vi "Tell Forward Self.vi"(6 "Msg":refnum<class "Msg.lvclass">, 7 "Actor in":refnum<class "Actor.lvclass">, 9 "Msg DVR":refnum<data-value>) -> (0 "Error out":errorcluster, 5 "Actor out":refnum<class "Actor.lvclass">)   [LabVIEW 2020, in "jettl.lvlib"]
uses:
  jettl.lvlib
  Msg/Msg.lvclass
  Msg Contents/Msg Contents.lvclass
  Actor/Actor.lvclass
  Unified Actor Relation.ctl
  Teller.ctl
  Msg.ctl
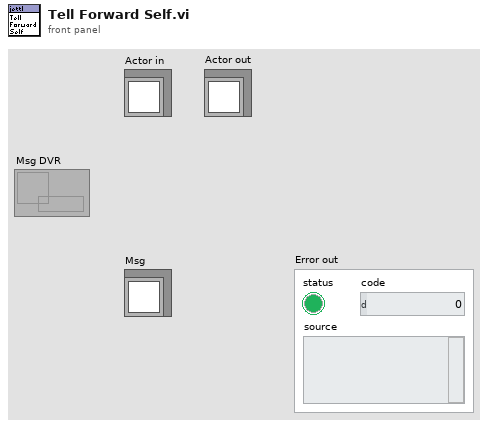
[diagram p1: front panel]
types:
  T1 = typedef "jettl.lvlib/Msg.ctl" = cluster{"Msg":refnum<class "Msg.lvclass">, "Msg Contents":refnum<class "Msg Contents.lvclass">, "Teller":T2}
  T2 = typedef "jettl.lvlib/Teller.ctl" = cluster{"Unified Actor Alias":string, "Unified Actor Relation":T3, "Absolute Time":timestamp, "Relative Time":dbl}
  T3 = typedef "jettl.lvlib/Unified Actor Relation.ctl" = enum16{"Self", "Parent", "Child"}
  T4 = typedef "jettl.lvlib/Unified Actor.ctl" = cluster{"Msgs":T5, "Leaf":bool, "Edge Actors":refnum<class "Actor.lvclass">[], "Mid Actors":refnum<class "Actor.lvclass">[], "Core Actors":refnum<class "Actor.lvclass">[], "Root":bool, "Alias":string, "UID":i32, "Transport":refnum<user-event>, "Address":refnum<event-registration>, "This VI":refnum<vi>}
  T5 = typedef "jettl.lvlib/Msgs.ctl" = cluster{"Inbound":T6, "Outbound":T6, "Implemented":T6, "Tell Init":T6, "Tell Init Self":T6, "Tell Init Parent":T6, "Tell Init Child":T6, "Tell Forward":T6, "Tell Forward Self":T6, "Tell Forward Parent":T6, "Tell Forward Child":T6}
  T6 = typedef "jettl.lvlib/Msg Set.ctl" = set{refnum<class "Msg.lvclass">}
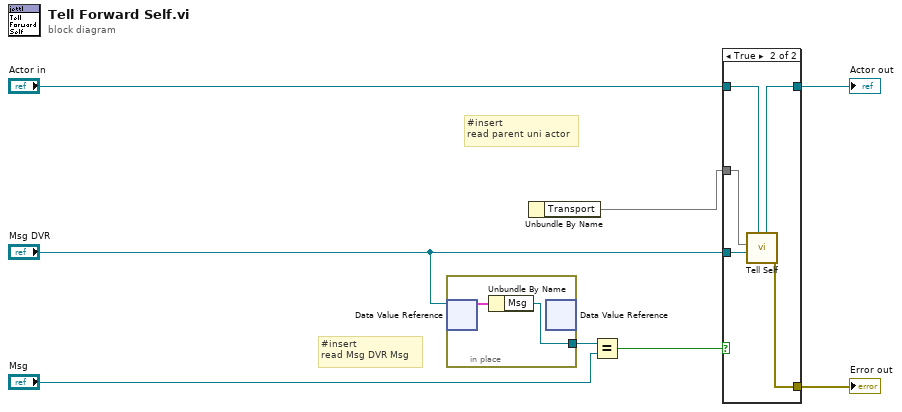
[diagram p0: block diagram]
diagram:
  # "#insert\nread Msg DVR Msg"
  # "#insert\nread parent uni actor"
  n1 = in-place {
    in-place-border: [w10] -> w5
    n2 = in-place-dvr #1("Msg DVR") -> (w11:T1)  [unwired: 1 out]
    n3 = Unbundle By Name(w11) -> ("Msg"=w10:refnum<class "Msg.lvclass">)
    n4 = in-place-dvr #1() -> ()  [unwired: 1 in, 2 out]
  }
  n5 = Unbundle By Name() -> (w2:T4, "Transport"=w1)
  n6 = Equal?(x=w5, y="Msg") -> (x = y?=w4:bool)
  n7 = case shown="True" w4 {
    tunnel: "Actor in" -> [w12 w16]
    tunnel: [_ w15] -> w9
    tunnel: [w12 w14] -> w8
    tunnel: "Msg DVR" -> [_ w17]
    tunnel: w1 -> [_ w13]
    frame False {
    }
    frame True {
      n8 = call "Tell Self.vi"("Actor in"=w16, "Msg DVR"=w17, "Transport"=w13) -> ("Error out"=w15:errorcluster, "Actor out"=w14:refnum<class "Actor.lvclass">)  [unwired: 7 in]
    }
  }
  "Error out" <- w9
  "Actor out" <- w8
